vi "Evaluate.vi"(8 "error in (no error)":errorcluster, 10 "Comparator":refnum<class "Comparator.lvclass">, 11 "One In":refnum<class "One.lvclass">) -> (0 "error out":errorcluster, 1 "Message":string, 2 "Passed?":bool)   [LabVIEW 2020, in "One.lvclass"]
uses:
  One.lvclass
  Core/Comparator/Comparator.lvclass
  One.lvclass/One.ctl
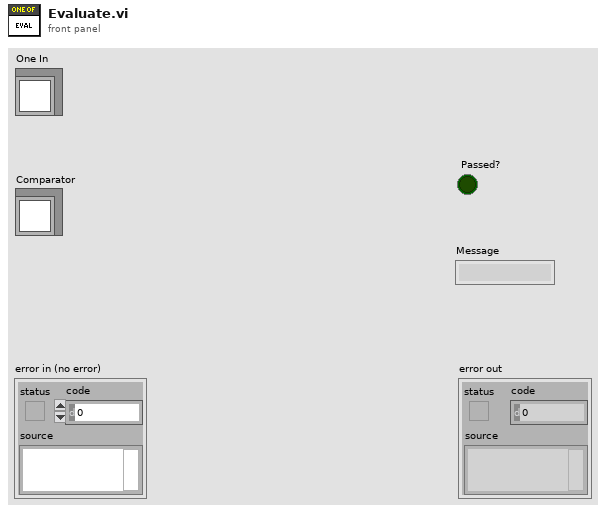
[diagram p1: front panel]
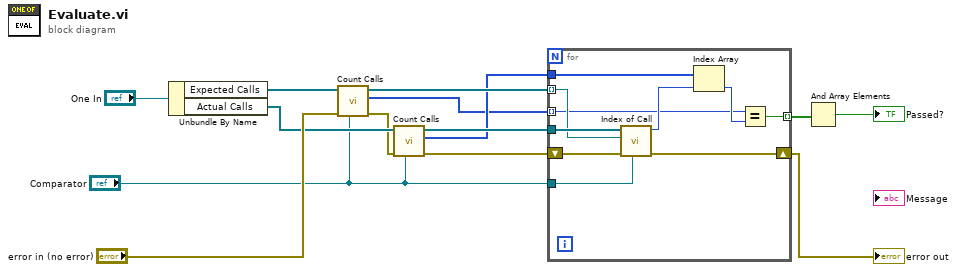
[diagram p0: block diagram]
diagram:
  n1 = Unbundle By Name("One In") -> ("Expected Calls"=w12:refnum<class "VI Call.lvclass">[], "Actual Calls"=w11:refnum<class "VI Call.lvclass">[])
  n2 = call "Count Calls.vi"("Comparator in"="Comparator", "error in (no error)"="error in (no error)", "Calls in"=w12) -> ("error out"=w10:errorcluster, "Call Count"=w4:i32[], "Unique Calls"=w8:refnum<class "VI Call.lvclass">[])  [unwired: 6 in]
  n3 = call "Count Calls.vi"("Comparator in"="Comparator", "error in (no error)"=w10, "Calls in"=w11) -> ("error out"=w7:errorcluster, "Call Count"=w5:i32[], "Unique Calls"=w9:refnum<class "VI Call.lvclass">[])  [unwired: 6 in]
  n4 = for {
    tunnel: w9 -> [w22]
    tunnel: w8 -> [w21] mode=indexing
    tunnel: "Comparator" -> [w15]
    shift-right: [w23] -> w6
    shift-left: w7 -> [w24]
    tunnel: w5 -> [w20]
    tunnel: w4 -> [w17] mode=indexing
    tunnel: [w16] -> w3 mode=indexing
    n5 = call "Index of Call.vi"("Comparator"=w15, "error in (no error)"=w24, "VI Call"=w21, "Unique Calls"=w22) -> ("error out"=w23:errorcluster, "f"=w19:i32)  [unwired: 6 in]
    n6 = Index Array(array=w20, index=w19) -> (element=w18:i32)
    n7 = Equal?(x=w17, y=w18) -> (x = y?=w16:bool)
  }
  "error out" <- w6
  n8 = And Array Elements(Boolean array=w3) -> (logical AND=→"Passed?":bool)
